vi "toml_example_dump.vi"(8 "error in (no error)":errorcluster) -> (0 "error out":errorcluster)   [LabVIEW 2017]
uses:
  40eee15b-28ef-4e74-a0ee-40500bcd5c6e.vi
  toml/toml_dump.vi
panel:
  out "toml":string
  in  "tables":T1
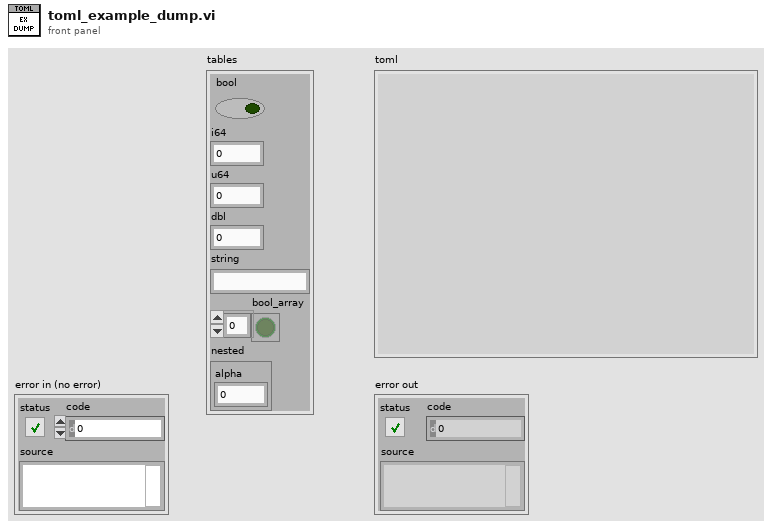
[diagram p1: front panel]
types:
  T1 = cluster{"bool":bool, "i64":i64, "u64":u64, "dbl":dbl, "string":string, "bool_array":bool[], "nested":cluster{"alpha":i32}}
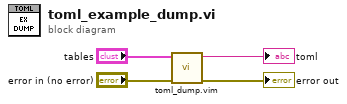
[diagram p0: block diagram]
diagram:
  n1 = call "toml_dump.vim"("error in (no error)"="error in (no error)", "tables"="tables") -> ("error out"=→"error out":errorcluster, "toml"=→"toml":string)  [unwired: 8 in]
